vi "ScanParam2DAQParam.vi"(8 "error in":errorcluster, 11 "AOL_Globals":T1={"Imaging Protocol"=enum."AOL Z-Stack", "Number of POI"=0, "Number of Miniscans"=0, "Number of Trials"=0, "Number of Cycles "=0, "# Averaged Frames"=0, "Laser power (%)"=0, "Pockels (V)"=0.0, "Acquisition Length (sec)"=0.0, "Fill time (us)"=0.0, "POI Dwell time (us)"=0.0, "Miniscan Dwell time per pixel (us)"=0.0, "PMT 1"=0.0, "PMT 2"=0.0, "Back Apperture (mA)"=200.0, "Frame Size"=0, "Center Frequency"=0.0, "Field of View (norm)"=0.0, "DwellTime (us)"=0.0, "Wavelength (nm)"=0.0, "Zoom"=0.0, "AOL Z"=0.0, "AOL Mode"=enum."Raster", "GridXY"=0.0, "GridZ"=0.0, "TriggerPeriod (sec)"=0.0, "Number of Pixels in Miniscan"=0, "Experiment folder path"=path "", "X centre"=0.0, "Y centre"=0.0, "Angle (degrees)"=0.0, "Plane Mode"=0, "Threshold"=[], "Regenerate Chirps"=FALSE, "Rectangle ROI length (pixels)"=0, "Rectangle ROI height (pixels)"=0, "AOD fill"=4900, "StartupDelay"=0, "Samples Wait after Trigger"=5080, "Slip Cycle"=600000, "Add Cycle"=TRUE, "Functional Mode"=enum."Point", "Z Start"=0.0, "Z Stop"=0.0, "# Planes"=0} {"Plane Mode" items=["XY Plane", "XZ Plane", "YZ Plane", "arbitraryplane"]; "Frame Size" items=["100X100"=100, "128X128"=128, "200X200"=200, "256X256"=256, "512X512"=512, "1024x1024"=1024, "2048x2048"=2048]; "Back Apperture (mA)" format="%#.6g"; "Pockels (V)" format="%#.6g"; "PMT 2" format="%#.6g"; "PMT 1" format="%#.6g"; "Angle (degrees)" format="%#.6g"; "POI Dwell time (us)" format="%#.6g"}) -> (0 "error out":errorcluster, 3 "DAQ Input Parameters(FlexRIO)":T7={"Mode"=enum."Scanning", "Zoom"=0, "Acceptance Angle"=0, "AOD fill"=0, "Wavelength"=0, "Speed of Sound(Va)"=0, "Samps-per-pix(P)"=0, "Numer-pixels-pointing(Np)"=0, "Samples Wait after Trigger"=0, "StartUp Delay"=0, "x-pixels-per-line(NPx) (fast)"=0, "y-pixels-per-line(NPy) (slow)"=0, "Repeat (Number of Cycles)"=0, "Number of Trials"=0, "Slip Cycle"=163840, "Use accumulate green"=FALSE, "Use accumulate red"=FALSE, "Add Cycle"=FALSE, "accn_noise"=6000.0, "var_y"=1.0, "var_x"=1.0, "New line trigger enabled"=FALSE} {"var_x" format="%#_14g"; "var_y" format="%#_14g"})   [LabVIEW 2017]
uses:
  Typedefs/Controls/DAQ Input Parameters(FlexRIO).ctl
  FPGA Host VIs/FPGA Typedefs/scan_typr.ctl
  Typedefs/Controls/AOL_Globals.ctl
  Typedefs/Imaging Protocols enum.ctl
  Typedefs/Frame Size.ctl
  Typedefs/AOL modes.ctl
  Typedefs/Plane Mode.ctl
  Typedefs/Functional Mode.ctl
panel:
  out "Number of Cycles":u64
  out "Repeat (Number of Cycles)":u32
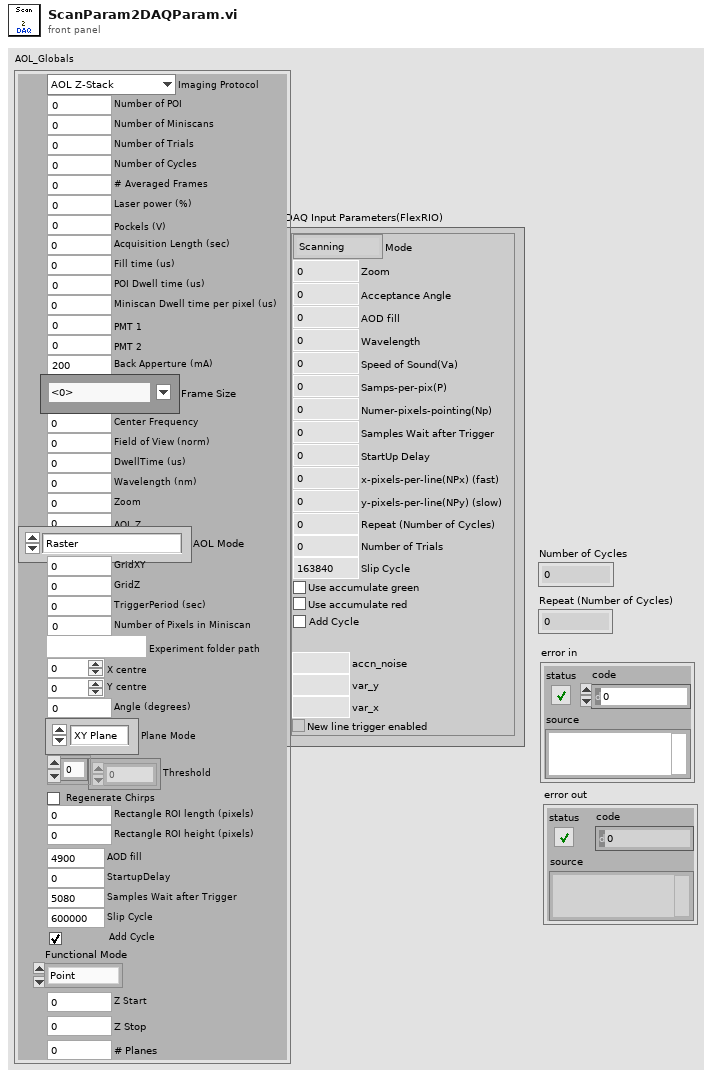
[diagram p1: front panel]
types:
  T1 = typedef "AOL_Globals.ctl" = cluster{"Imaging Protocol":T2, "Number of POI":u16, "Number of Miniscans":u16, "Number of Trials":u16, "Number of Cycles ":u64, "# Averaged Frames":u16, "Laser power (%)":u8, "Pockels (V)":dbl, "Acquisition Length (sec)":dbl, "Fill time (us)":dbl, "POI Dwell time (us)":dbl, "Miniscan Dwell time per pixel (us)":dbl, "PMT 1":dbl, "PMT 2":dbl, "Back Apperture (mA)":dbl, "Frame Size":T3, "Center Frequency":dbl, "Field of View (norm)":dbl, "DwellTime (us)":dbl, "Wavelength (nm)":dbl, "Zoom":dbl, "AOL Z":dbl, "AOL Mode":T4, "GridXY":dbl, "GridZ":dbl, "TriggerPeriod (sec)":dbl, "Number of Pixels in Miniscan":u16, "Experiment folder path":path, "X centre":dbl, "Y centre":dbl, "Angle (degrees)":dbl, "Plane Mode":T5, "Threshold":u16[], "Regenerate Chirps":bool, "Rectangle ROI length (pixels)":u16, "Rectangle ROI height (pixels)":u16, "AOD fill":u16, "StartupDelay":i32, "Samples Wait after Trigger":u16, "Slip Cycle":u32, "Add Cycle":bool, "Functional Mode":T6, "Z Start":dbl, "Z Stop":dbl, "# Planes":i32}
  T2 = typedef "Imaging Protocols enum.ctl" = enum16{"AOL Z-Stack", "Motor Z Stack", "Functional Acquisition", "Single Plane Acquisition", "Volume Acquisition", "Live Imaging", "Live Plane Imaging", "Live Volume Imaging"}
  T3 = typedef "Frame Size.ctl" = u16
  T4 = typedef "AOL modes.ctl" = enum16{"Raster", "Structural", "Pointing", "Mini Scan", "Alignment"}
  T5 = typedef "Plane Mode.ctl" = u16
  T6 = typedef "Functional Mode.ctl" = enum16{"Point", "Line", "Patch", "Plane", "Volume"}
  T7 = typedef "DAQ Input Parameters(FlexRIO).ctl" = cluster{"Mode":T8, "Zoom":i8, "Acceptance Angle":i8, "AOD fill":u16, "Wavelength":i16, "Speed of Sound(Va)":i8, "Samps-per-pix(P)":i16, "Numer-pixels-pointing(Np)":u32, "Samples Wait after Trigger":u16, "StartUp Delay":i32, "x-pixels-per-line(NPx) (fast)":u16, "y-pixels-per-line(NPy) (slow)":u16, "Repeat (Number of Cycles)":u32, "Number of Trials":u16, "Slip Cycle":u32, "Use accumulate green":bool, "Use accumulate red":bool, "Add Cycle":bool, "accn_noise":fxp<+,16,16>, "var_y":fxp<+,16,4>, "var_x":fxp<+,16,4>, "New line trigger enabled":bool}
  T8 = typedef "scan_typr.ctl" = enum16{"Scanning", "Pointing", "Pointing & MC", "Scanning & MC"}
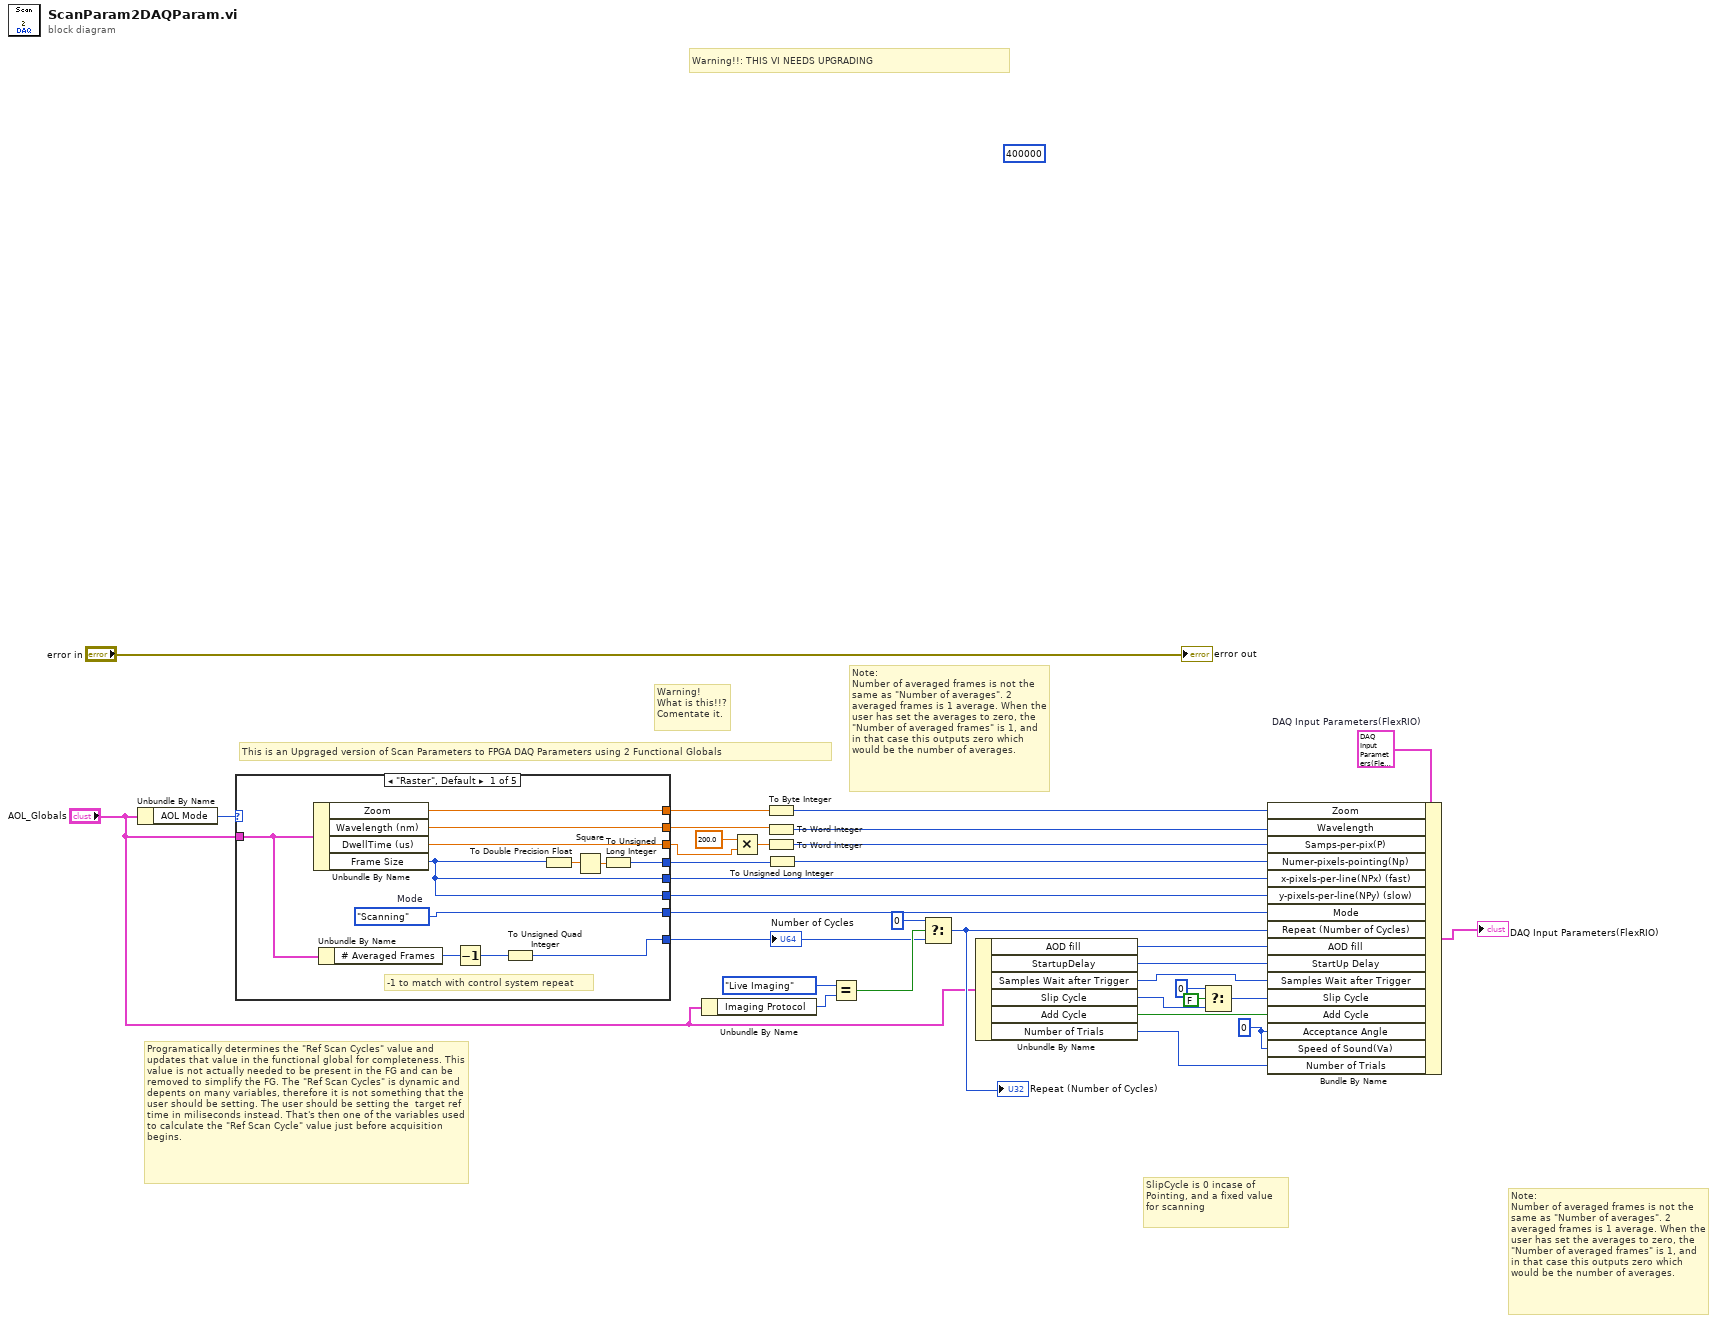
[diagram p0: block diagram]
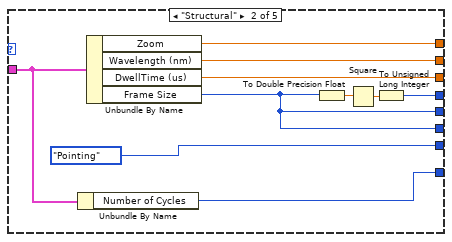
[diagram p2: hidden frame]
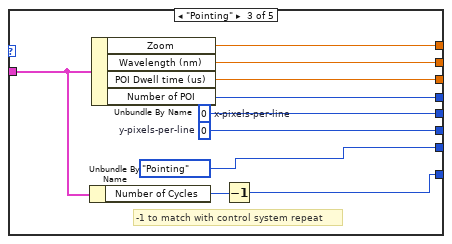
[diagram p3: hidden frame]
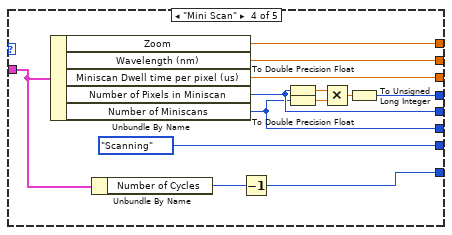
[diagram p4: hidden frame]
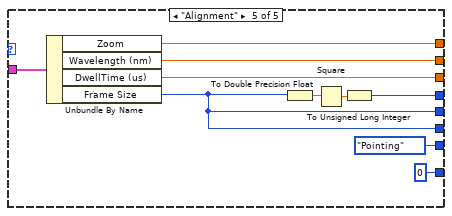
[diagram p5: hidden frame]
diagram:
  w3 = i8 0 ("Speed of Sound(Va)")
  w8 = T7 {"Mode"=enum."Scanning", "Zoom"=0, "Acceptance Angle"=0, "AOD fill"=0, "Wavelength"=0, "Speed of Sound(Va)"=0, "Samps-per-pix(P)"=0, "Numer-pixels-pointing(Np)"=0, "Samples Wait after Trigger"=0, "StartUp Delay"=0, "x-pixels-per-line(NPx) (fast)"=0, "y-pixels-per-line(NPy) (slow)"=0, "Repeat (Number of Cycles)"=0, "Number of Trials"=0, "Slip Cycle"=163840, "Use accumulate green"=FALSE, "Use accumulate red"=FALSE, "Add Cycle"=FALSE, "accn_noise"=6000.0, "var_y"=1.0, "var_x"=1.0, "New line trigger enabled"=FALSE}  # DAQ Input Parameters(FlexRIO)
  (unwired) 400000 ("Ref Scan Cycles")
  # "Programatically determines the \"Ref Scan Cycles\" value and updates that value in the functional global for completeness. This value is not actually needed to be present in the FG and can be removed to simplify the FG. The \"Ref Scan Cycles\" is dynamic and depents on many variables, therefore it is not something that the user should be setting. The user should be setting the  target ref time in miliseconds instead. That's then one of the variables used to calculate the \"Ref Scan Cycle\" value just before acquisition begins."
  # "Warning!\nWhat is this!!?\nComentate it."
  # "Note:\nNumber of averaged frames is not the same as \"Number of averages\". 2 averaged frames is 1 average. When the user has set the averages to zero, the \"Number of averaged frames\" is 1, and in that case this outputs zero which would be the number of averages."
  # "SlipCycle is 0 incase of Pointing, and a fixed value for scanning"
  # "Note:\nNumber of averaged frames is not the same as \"Number of averages\". 2 averaged frames is 1 average. When the user has set the averages to zero, the \"Number of averaged frames\" is 1, and in that case this outputs zero which would be the number of averages."
  # "This is an Upgraged version of Scan Parameters to FPGA DAQ Parameters using 2 Functional Globals"
  # "Warning!!: THIS VI NEEDS UPGRADING"
  n1 = Unbundle By Name("AOL_Globals") -> ("AOL Mode"=w34:T4)
  n2 = case shown="\"Raster\", Default" w34 {
    tunnel: "AOL_Globals" -> [w39 w49 w61 w75 w89]
    tunnel: [w46 w56 w66 w79 w88] -> w33
    tunnel: [w45 w55 w65 w78 w87] -> w28
    tunnel: [w41 w51 w59 w76 w83] -> w23
    tunnel: [w42 w52 w64 w77 w84] -> w22
    tunnel: [w40 w50 w63 w72 w82] -> w26
    tunnel: [w40 w50 w62 w71 w82] -> w25
    tunnel: [w35 scan_typr."Pointing" ("Mode") scan_typr."Pointing" ("Mode") scan_typr."Scanning" ("Mode") scan_typr."Pointing" ("Mode")] -> w20
    tunnel: [w36 w48 w58 w70 u64 0 ("Number of Cycles")] -> w16
    frame "Raster", Default {
      w35 = scan_typr."Scanning"  # Mode
      # "-1 to match with control system repeat"
      n3 = Unbundle By Name(w39) -> ("Zoom"=w46:dbl, "Wavelength (nm)"=w42:dbl, "DwellTime (us)"=w45:dbl, "Frame Size"=w40:T3)
      n4 = Unbundle By Name(w39) -> ("# Averaged Frames"=w38:u16)
      n5 = Decrement(x=w38) -> (x-1=w37:u16)
      n6 = To Unsigned Quad Integer(1:w37) -> (0:w36:u64)
      n7 = To Double Precision Float(number=w40) -> (double precision float=w44:dbl)
      n8 = Square(x=w44) -> (x^2=w43:dbl)
      n9 = To Unsigned Long Integer(number=w43) -> (unsigned 32bit integer=w41:u32)
    }
    frame "Structural" {
      n10 = Unbundle By Name(w49) -> ("Number of Cycles"=w48:u64)
      n11 = Unbundle By Name(w49) -> ("Zoom"=w56:dbl, "Wavelength (nm)"=w52:dbl, "DwellTime (us)"=w55:dbl, "Frame Size"=w50:T3)
      n12 = To Double Precision Float(number=w50) -> (double precision float=w54:dbl)
      n13 = Square(x=w54) -> (x^2=w53:dbl)
      n14 = To Unsigned Long Integer(number=w53) -> (unsigned 32bit integer=w51:u32)
    }
    frame "Pointing" {
      w62 = u16 0  # y-pixels-per-line
      w63 = u16 0  # x-pixels-per-line
      # "-1 to match with control system repeat"
      n15 = Unbundle By Name(w61) -> ("Number of Cycles"=w60:u64)
      n16 = Unbundle By Name(w61) -> ("Zoom"=w66:dbl, "Wavelength (nm)"=w64:dbl, "POI Dwell time (us)"=w65:dbl, "Number of POI"=w59:u16)
      n17 = Decrement(x=w60) -> (x-1=w58:u64)
    }
    frame "Mini Scan" {
      n18 = Unbundle By Name(w75) -> ("Zoom"=w79:dbl, "Wavelength (nm)"=w77:dbl, "Miniscan Dwell time per pixel (us)"=w78:dbl, "Number of Pixels in Miniscan"=w72:u16, "Number of Miniscans"=w71:u16)
      n19 = Unbundle By Name(w75) -> ("Number of Cycles"=w74:u64)
      n20 = Decrement(x=w74) -> (x-1=w70:u64)
      n21 = To Double Precision Float(number=w72) -> (double precision float=w69:dbl)
      n22 = To Double Precision Float(number=w71) -> (double precision float=w68:dbl)
      n23 = Multiply(x=w69, y=w68) -> (x*y=w73:dbl)
      n24 = To Unsigned Long Integer(number=w73) -> (unsigned 32bit integer=w76:u32)
    }
    frame "Alignment" {
      n25 = Unbundle By Name(w89) -> ("Zoom"=w88:dbl, "Wavelength (nm)"=w84:dbl, "DwellTime (us)"=w87:dbl, "Frame Size"=w82:T3)
      n26 = To Double Precision Float(number=w82) -> (double precision float=w86:dbl)
      n27 = Square(x=w86) -> (x^2=w85:dbl)
      n28 = To Unsigned Long Integer(number=w85) -> (unsigned 32bit integer=w83:u32)
    }
  }
  "Number of Cycles" <- w16
  n29 = Unbundle By Name("AOL_Globals") -> ("Imaging Protocol"=w15:T2)
  n30 = Multiply(x=200.0, y=w28) -> (x*y=w31:dbl)
  n31 = To Byte Integer(number=w33) -> (8bit integer=w32:i8)
  n32 = To Word Integer(number=w22) -> (16bit integer=w27:i16)
  n33 = To Word Integer(number=w31) -> (16bit integer=w29:i16)
  n34 = To Unsigned Long Integer(number=w23) -> (unsigned 32bit integer=w24:u32)
  n35 = Equal?(x=Imaging_Protocols_enum."Live Imaging", y=w15) -> (x = y?=w17:bool)
  n36 = Select(t=u64 0, s=w17, f=w16) -> (s? t:f=w12:u64)
  "Repeat (Number of Cycles)" <- w12
  n37 = Unbundle By Name("AOL_Globals") -> ("AOD fill"=w7:u16, "StartupDelay"=w11:i32, "Samples Wait after Trigger"=w6:u16, "Slip Cycle"=w5:u32, "Add Cycle"=w10:bool, "Number of Trials"=w1:u16)
  n38 = Select(t=u32 0, s=FALSE, f=w5) -> (s? t:f=w4:u32)
  n39 = Bundle By Name(cluster=w8, "Zoom"=w32, "Wavelength"=w27, "Samps-per-pix(P)"=w29, "Numer-pixels-pointing(Np)"=w24, "x-pixels-per-line(NPx) (fast)"=w26, "y-pixels-per-line(NPy) (slow)"=w25, "Mode"=w20, "Repeat (Number of Cycles)"=w12, "AOD fill"=w7, "StartUp Delay"=w11, "Samples Wait after Trigger"=w6, "Slip Cycle"=w4, "Add Cycle"=w10, "Acceptance Angle"=w3, "Speed of Sound(Va)"=w3, "Number of Trials"=w1) -> (→"DAQ Input Parameters(FlexRIO)":T7)
  "error out" <- "error in"
